vi "SystemManager_LV2009.vi"() -> ()   [LabVIEW 2009]
panel:
  in  "stop":bool
  in  "SystemMonitor":refnum<k7>(container)
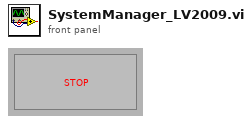
[diagram p1: front panel]
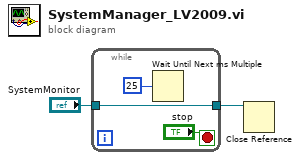
[diagram p0: block diagram]
diagram:
  n1 = while {
    tunnel: "SystemMonitor" -> [w5]
    tunnel: [w5] -> w2
    stop <- "stop" stop-if-true
    n2 = Wait Until Next ms Multiple(millisecond multiple=u32 25) -> ()  [unwired: 1 out]
  }
  n3 = Close Reference(reference=w2) -> ()  [unwired: 1 in, 1 out]
